vi "SD-Read Registry Value DWORD.vi"(8 "error in (no error)":errorcluster, 9 "default data":u32, 10 "value":string, 11 "refnum":T1) -> (0 "error out":errorcluster, 1 "DWORD data":u32, 2 "data type":T2(ring), 3 "refnum out":T1)   [LabVIEW 2020]
doc: "Reads data and data type from value. If the key or value does not exist or an unrecoverable error occurs, the VI returns the default value."
uses:
  SD-Registry refnum.ctl
  Advapi32.dll
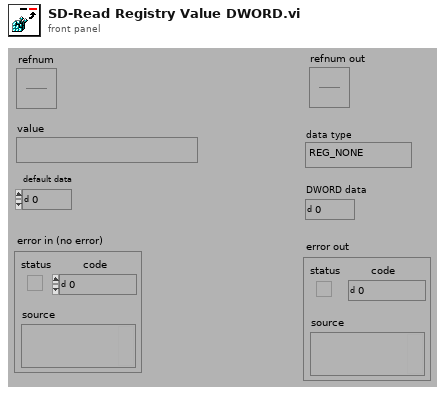
[diagram p1: front panel]
types:
  T1 = typedef "SD-Registry refnum.ctl" = refnum<k1>
  T2 = enum32{"REG_NONE", "REG_SZ", "REG_EXPAND_SZ", "REG_BINARY", "REG_DWORD_LITTLE_ENDIAN", "REG_DWORD_BIG_ENDIAN", "REG_LINK", "REG_MULTI_SZ", "REG_RESOURCE_LIST", "REG_FULL_RESOURCE_DESCRIPTOR", "REG_RESOURCE_REQUIREMENTS_LIST"}
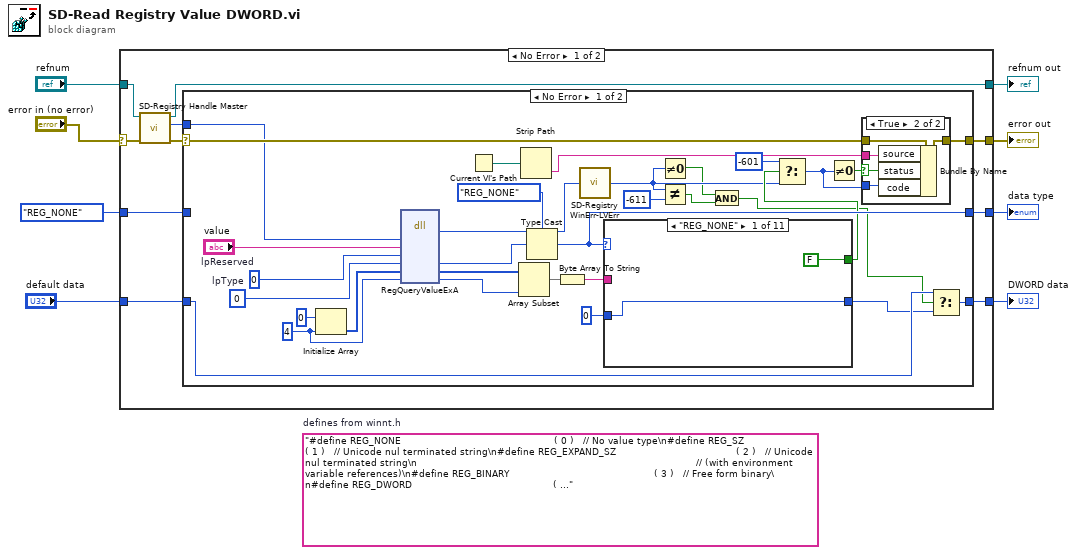
[diagram p0: block diagram]
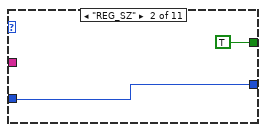
[diagram p3: hidden frame]
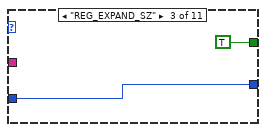
[diagram p4: hidden frame]
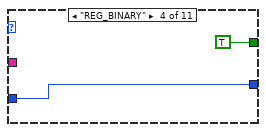
[diagram p5: hidden frame]
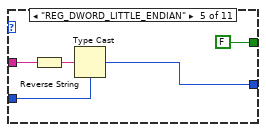
[diagram p6: hidden frame]
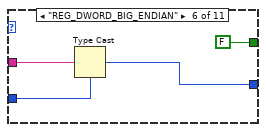
[diagram p7: hidden frame]
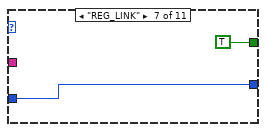
[diagram p8: hidden frame]
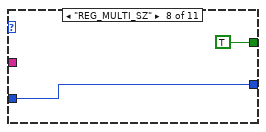
[diagram p9: hidden frame]
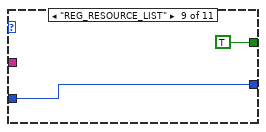
[diagram p10: hidden frame]
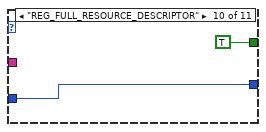
[diagram p11: hidden frame]
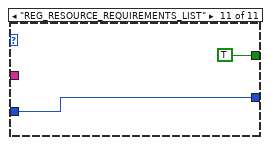
[diagram p12: hidden frame]
diagram:
  (unwired) "#define REG_NONE                                                   ( 0 )   // No value type\n#define REG_SZ                                                        ( 1 )   // Unicode nul terminated string\n#define REG_EXPAND_SZ                                        ( 2 )   // Unicode nul terminated string\n                                                                                             // (with environment variable references)\n#define REG_BINARY                                                ( 3 )   // Free form binary\n#define REG_DWORD                                               ( 4 )   // 32-bit number\n#define REG_DWORD_LITTLE_ENDIAN                  ( 4 )   // 32-bit number (same as REG_DWORD)\n#define REG_DWORD_BIG_ENDIAN                        ( 5 )   // 32-bit number\n#define REG_LINK                                                      ( 6 )   // Symbolic Link (unicode)\n#define REG_MULTI_SZ                                            ( 7 )   // Multiple Unicode strings\n#define REG_RESOURCE_LIST                                ( 8 )   // Resource list in the resource map\n#define REG_FULL_RESOURCE_DESCRIPTOR      ( 9 )   // Resource list in the hardware description\n#define REG_RESOURCE_REQUIREMENTS_LIST ( 10 )\n"  # defines from winnt.h
  n1 = case shown="No Error" "error in (no error)" {
    selector: "error in (no error)" -> [w15 w90]
    tunnel: [w18 w88] -> w7
    tunnel: [w17 w87] -> w8
    tunnel: [w16 w90] -> w6
    tunnel: "refnum" -> [w14 w89]
    tunnel: [w13 w89] -> w3
    tunnel: T2."REG_NONE" -> [w10 w88]
    tunnel: "default data" -> [w9 w87]
    frame No Error {
      n2 = call "SD-Registry Handle Master.vi"("error in (no error)"=w15, "refnum"=w14) -> ("error out"=w11:errorcluster, "key handle out"=w12:u64, "refnum out"=w13:T1)  [unwired: 4 in, 3 out]
      n3 = case shown="No Error" w11 {
        selector: w11 -> [w38 w86]
        tunnel: [w50 w85] -> w18
        tunnel: [w36 w84] -> w17
        tunnel: [w44 w86] -> w16
        tunnel: w12 -> [w25 _]
        tunnel: w10 -> [_ w85]
        tunnel: w9 -> [w35 w84]
        frame No Error {
          w28 = u32 0  # lpType
          w29 = u32 4
          w27 = u64 0  # lpReserved
          n4 = Initialize Array(u8 0, w29) -> (w21:u8[])
          n5 = dll-call lib="Advapi32.dll" fn="RegQueryValueExA"("hKey"=w25, "lpValueName"="value", "lpReserved"=w27, "lpType"=w28, "lpData"=w21, "lpcbData"=w29) -> ("return type"=w19:i32, "lpType"=w24:u32, "lpData"=w22:u8[], "lpcbData"=w23:u32)  [unwired: 5 in, 3 out]
          n6 = Current VI's Path() -> (path=w46:path)
          n7 = Array Subset(array=w22, length=w23) -> (w45:u8[])  [unwired: 1 in]
          n8 = Strip Path(path=w46) -> (name=w47:string)  [unwired: 1 out]
          n9 = Type Cast(type=T2."REG_NONE", x=w24) -> (*(type *) &x=w50:T2)
          n10 = Byte Array To String(unsigned byte array=w45) -> (string=w43:string)
          n11 = call "SD-Registry WinErr-LVErr.vi"("Windows error"=w19) -> ("LabVIEW error"=w37:i32)  [unwired: 4 out]
          n12 = case shown="\"REG_NONE\"" w50 {
            tunnel: w43 -> [_ _ _ _ w69 w73 _ _ _ _ _]
            tunnel: [w58 w60 w62 w64 w68 w72 w75 w77 w79 w81 w83] -> w34
            tunnel: u32 0 -> [w58 w60 w62 w64 w67 w71 w75 w77 w79 w81 w83]
            tunnel: [FALSE TRUE TRUE TRUE FALSE FALSE TRUE TRUE TRUE TRUE TRUE] -> w41
            frame "REG_NONE" {
            }
            frame "REG_SZ" {
            }
            frame "REG_EXPAND_SZ" {
            }
            frame "REG_BINARY" {
            }
            frame "REG_DWORD_LITTLE_ENDIAN" {
              n13 = Reverse String(1:w69) -> (0:w66:string)
              n14 = Type Cast(type=w67, x=w66) -> (*(type *) &x=w68:u32)
            }
            frame "REG_DWORD_BIG_ENDIAN" {
              n15 = Type Cast(type=w71, x=w73) -> (*(type *) &x=w72:u32)
            }
            frame "REG_LINK" {
            }
            frame "REG_MULTI_SZ" {
            }
            frame "REG_RESOURCE_LIST" {
            }
            frame "REG_FULL_RESOURCE_DESCRIPTOR" {
            }
            frame "REG_RESOURCE_REQUIREMENTS_LIST" {
            }
          }
          n16 = Not Equal To 0?(x=w37) -> (x != 0?=w31:bool)
          n17 = Not Equal?(x=w37, y=-611) -> (x != y?=w32:bool)
          n18 = And(x=w31, y=w32) -> (x .and. y?=w30:bool)
          n19 = Select(t=-601, s=w41, f=w37) -> (s? t:f=w42:i32)
          n20 = Not Equal To 0?(x=w42) -> (x != 0?=w39:bool)
          n21 = case shown="True" w39 {
            selector: w39 -> [_ w52]
            tunnel: w47 -> [_ w56]
            tunnel: w38 -> [w51 w55]
            tunnel: [w51 w54] -> w44
            tunnel: w42 -> [_ w53]
            frame False {
            }
            frame True {
              n22 = Bundle By Name(cluster=w55, "source"=w56, "status"=w52, "code"=w53) -> (w54:errorcluster)
            }
          }
          n23 = Select(t=w35, s=w30, f=w34) -> (s? t:f=w36:u32)
        }
        frame Error {
        }
      }
    }
    frame Error {
    }
  }
  "error out" <- w6
  "DWORD data" <- w8
  "data type" <- w7
  "refnum out" <- w3
